vi "test.ingest_video 2.vi"() -> ()   [LabVIEW 2020]
uses:
  Nominal Client/datasources/dataset/dataset.lvclass
  nominal types/channelConfig/channelConfig.lvclass
  Nominal Client/Nominal Client.lvclass/Nominal Client.ctl
  nominal types/workspace/workspace.lvclass/workspace.ctl
  ae172e34-dffc-4b12-83ea-48ef3a2c3c44.vi
  f68fde30-30e4-4b08-97bf-6f7da0132bc9.vi
  d999190f-fee9-49b3-afb9-f232f2b660b8.vi
  Nominal Client/private_data.set.vi
  nominal types/workspace/id.get.vi
  nominal types/workspace/rid.get.vi
  <vilib>/AdvancedString/1D String Array to Delimited String.vi
  Nominal Client/workspace.set.vi
  nominal types/timestampManifest/noManifest/noManifest.lvclass
  C:/code/labview-client/lv_src/nominal types/timestampManifest/timestampManifest/timestampManifest.lvclass
  Nominal Client/datasources/s3/s3.lvclass
  C:/code/labview-client/lv_src/Nominal Client/datasources/source/source.lvclass
  <vilib>/Utility/error.llb/Error Cluster From Error Code.vi
  <vilib>/addons/_JKI.lib/REST Client/classes/REST Client/Create REST Client.vi
  reqwest/NewHttpSession.vi
  Nominal Client/workspace_cache.get_from_rid.vi
  Nominal Client/workspace_cache.get.vi
  Nominal Client/datasources/target/create_new.vi
  Nominal Client/datasources/source/create_s3.vi
  nominal types/timestampManifest/create.noManifest_scale_factor.vi
  Nominal Client/ingest_video.vi
  Nominal Client/video.get_ingest_status.vi
  reqwest/DestroyHttpSession.vi
  Nominal Client/Nominal Client.lvclass
  nominal types/workspace/workspace.lvclass
  <vilib>/addons/_JKI.lib/REST Client/classes/REST Client/REST Client.lvclass
  reqwest/reQwestClient.lvclass
  Nominal Client/datasources/source/source.lvclass
  Nominal Client/datasources/target/target.lvclass
  nominal types/timestampManifest/timestampManifest.lvlib
  C:/code/labview-client/lv_src/Nominal Client/datasources/payload/payload.lvclass
  C:/code/labview-client/lv_src/nominal types/timestampManifest/noManifest/noManifest.lvclass
  C:/code/labview-client/lv_src/Nominal Client/datasources/s3/s3.lvclass
panel:
  out "Progress":dbl(slide) scale=0.0..1.0
  out "unsigned byte array":u8[](array[numeric]) format="%08b"
  out "Status":string
  out "Response":string
  out "datasetFileId":string
  out "datasetRid":string
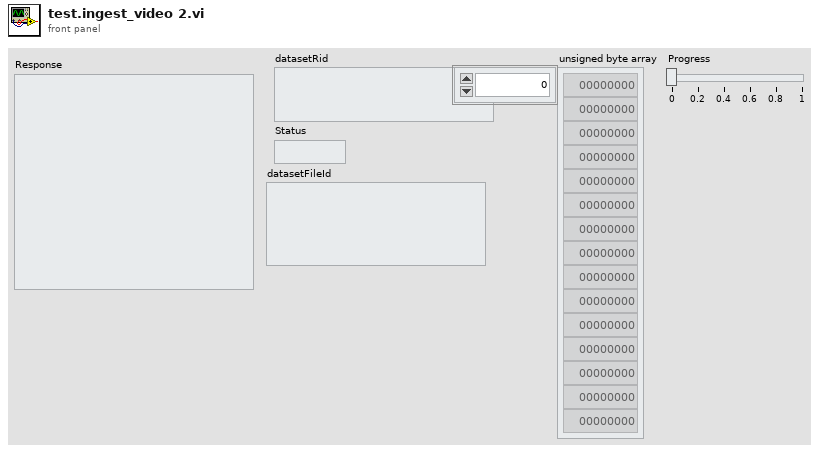
[diagram p1: front panel]
types:
  T1 = cluster{"dataset":refnum<class "dataset.lvclass">, "channelConfig":refnum<class "channelConfig.lvclass">}
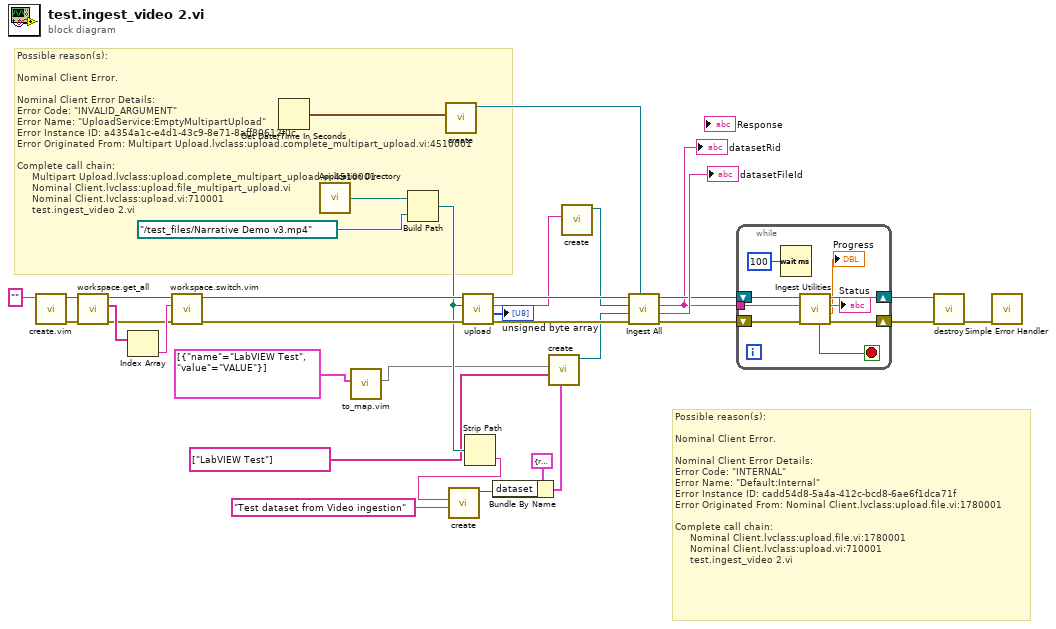
[diagram p0: block diagram]
diagram:
  # "Possible reason(s):\n\nNominal Client Error.\n\nNominal Client Error Details:\nError Code: \"INVALID_ARGUMENT\"\nError Name: \"UploadService:EmptyMultipartUpload\"\nError Instance ID: a4354a1c-e4d1-43c9-8e71-8aff80612f0c\nError Originated From: Multipart Upload.lvclass:upload.complete_multipart_upload.vi:4510001\n\nComplete call chain:\n     Multipart Upload.lvclass:upload.complete_multipart_upload.vi:4510001\n     Nominal Client.lvclass:upload.file_multipart_upload.vi\n     Nominal Client.lvclass:upload.vi:710001\n     test.ingest_video 2.vi"
  # "Possible reason(s):\n\nNominal Client Error.\n\nNominal Client Error Details:\nError Code: \"INTERNAL\"\nError Name: \"Default:Internal\"\nError Instance ID: cadd54d8-5a4a-412c-bcd8-6ae6f1dca71f\nError Originated From: Nominal Client.lvclass:upload.file.vi:1780001\n\nComplete call chain:\n     Nominal Client.lvclass:upload.file.vi:1780001\n     Nominal Client.lvclass:upload.vi:710001\n     test.ingest_video 2.vi"
  n1 = call "create.vim"("API Token (string or path)"="") -> ("error out"=w23:errorcluster, "Nominal Client"=w27:refnum<class "Nominal Client.lvclass">)  [unwired: 9 in]
  n2 = call "workspace.get_all.vi"("error in"=w23, "Nominal Client in"=w27) -> ("error out"=w22:errorcluster, "Workspace RIDs"=w25:string[], "Nominal Client out"=w26:refnum<class "Nominal Client.lvclass">)  [unwired: 5 in, 2 out]
  n3 = Index Array(array=w25) -> (element=w24:string)  [unwired: 1 in]
  n4 = call "workspace.switch.vim"("error in"=w22, "Workspace RID (string or path)"=w24, "Nominal Client in"=w26) -> ("error out"=w21:errorcluster, "Nominal Client out"=w20:refnum<class "Nominal Client.lvclass">)  [unwired: 7 in]
  n5 = Get Date/Time In Seconds() -> (seconds since 1Jan1904=w2:timestamp)
  n6 = call <vilib>:"Application Directory.vi"() -> ("Application Directory"=w29:path)
  n7 = call "to_map.vim"("Map"=cluster{"name":string, "value":string}[] [{"name"="LabVIEW Test", "value"="VALUE"}] ("properties")) -> ("Map out"=w11:map{string, string})  [unwired: 10 in]
  n8 = Build Path(base path=w29, name or relative path=path "../test_files/Narrative Demo v3.mp4") -> (appended path=w15:path)
  n9 = call-poly "create.vi"("startingTimestamp"=w2) -> ("Timestamp Manifest"=w3:refnum<class "noManifest.lvclass">)  [unwired: 10 in]
  n10 = call "upload.vi"("error in"=w21, "File"=w15, "Nominal Client in"=w20) -> ("error out"=w34:errorcluster, "unsigned byte array"=→"unsigned byte array":u8[], "Path to S3 File"=w33:string, "Nominal Client out"=w35:refnum<class "Nominal Client.lvclass">)  [unwired: 5 in]
  n11 = Strip Path(path=w15) -> (name=w14:string)  [unwired: 1 out]
  n12 = call "create.vi"("Description"="Test dataset from Video ingestion", "Name"=w14) -> ("dataset"=w17:refnum<class "dataset.lvclass">)  [unwired: 9 in]
  n13 = Bundle By Name(cluster=T1 {"dataset"=refnum, "channelConfig"=refnum} ("Optional"), "dataset"=w17) -> (w18:T1)
  n14 = call-poly "create.vi"("Optional"=w18, "Labels"=string[] ["LabVIEW Test"] ("labels"), "Properties"=w11) -> ("New Target"=w31:refnum<class "target.lvclass">)  [unwired: 8 in]
  n15 = call-poly "create.vi"("Path"=w33) -> ("source"=w32:refnum<class "s3.lvclass">)  [unwired: 10 in]
  n16 = call-poly "Ingest All.vi"("Timestamp Manifest"=w3, "error in"=w34, "Target"=w31, "Source"=w32, "Nominal Client in"=w35) -> ("error out"=w7:errorcluster, "videoFileRid"=→"datasetFileId":string, "videoRid"=w6:string, "Nominal Client out"=w8:refnum<class "Nominal Client.lvclass">)  [unwired: 3 in]
  "datasetRid" <- w6
  n17 = while {
    tunnel: w6 -> [w42]
    shift-right: [w41] -> w4
    shift-left: w8 -> [w44]
    shift-right: [w40] -> w5
    shift-left: w7 -> [w43]
    stop <- w36 stop-if-true
    n18 = Wait (ms)(milliseconds to wait=u32 100) -> ()  [unwired: 1 out]
    n19 = call-poly "Ingest Utilities.vi"("error in"=w43, "Video RID"=w42, "Nominal Client in"=w44) -> ("error out"=w40:errorcluster, "Progress (0-1)"=→"Progress":dbl, "Status"=→"Status":string, "Nominal Client out"=w41:refnum<class "Nominal Client.lvclass">, "Complete"=w36:bool)  [unwired: 4 in]
  }
  n20 = call "destroy.vi"("error in"=w5, "Nominal Client"=w4) -> ("error out"=w10:errorcluster)  [unwired: 9 in]
  n21 = call <vilib>:"Simple Error Handler.vi"("error in (no error)"=w10) -> ()  [unwired: 4 in, 5 out]
